vi "intMultiply.vi"(8 "Error in (no error)":errorcluster, 10 "Int2 in":refnum<class "IntClass.lvclass">, 11 "Int1 in":refnum<class "IntClass.lvclass">) -> (0 "Error out":errorcluster, 1 "Timing":u32, 3 "Int1 * Int2":refnum<class "IntClass.lvclass">)   [LabVIEW 2011, in "IntClass.lvclass"]
uses:
  IntClass.lvclass
  IntClass.lvclass/IntClass.ctl
  UintClass/UintClass.lvclass
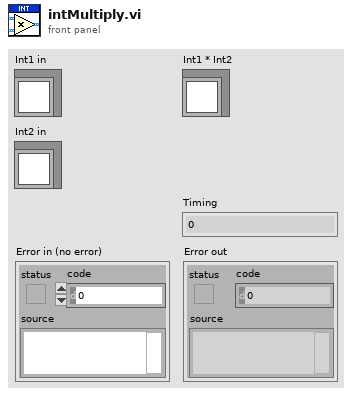
[diagram p1: front panel]
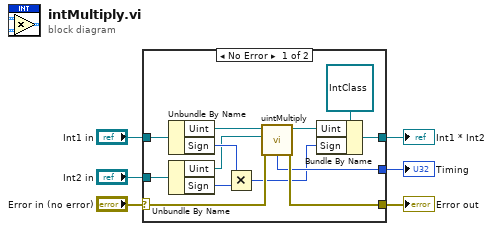
[diagram p0: block diagram]
diagram:
  n1 = case shown="No Error" "Error in (no error)" {
    selector: "Error in (no error)" -> [w17 w20]
    tunnel: "Int1 in" -> [w19 _]
    tunnel: "Int2 in" -> [w18 _]
    tunnel: [w16 w20] -> w3
    tunnel: [w15 _] -> w2
    tunnel: [w14 _] -> w1
    frame No Error {
      n2 = Unbundle By Name(w19) -> ("Uint"=w11:refnum<class "UintClass.lvclass">, "Sign"=w12:i8)
      n3 = Unbundle By Name(w18) -> ("Uint"=w10:refnum<class "UintClass.lvclass">, "Sign"=w13:i8)
      n4 = Multiply(x=w12, y=w13) -> (x*y=w9:i8)
      n5 = call "uintMultiply.vi"("Error in (no error)"=w17, "Uint2 in"=w10, "Uint1 in"=w11) -> ("Error out"=w16:errorcluster, "Timing"=w14:u32, "Uint1 * Uint2"=w8:refnum<class "UintClass.lvclass">)  [unwired: 6 in]
      n6 = Bundle By Name(cluster=refnum<class "IntClass.lvclass"> refnum ("Int1 in"), "Uint"=w8, "Sign"=w9) -> (w15:refnum<class "IntClass.lvclass">)
    }
    frame Error {
    }
  }
  "Int1 * Int2" <- w2
  "Error out" <- w3
  "Timing" <- w1
